vi "FPGA_frame.vi"(8 "error in":errorcluster) -> (0 "error out":errorcluster)   [LabVIEW 2010]
uses:
  fpgaVIsAndControls/DDS_board_init_cluster.ctl
  fpgaVIsAndControls/FPGA_parameters_cluster.ctl
  common_typedefs/channels_cluster.ctl
  fpgaVIsAndControls/scan_point_cluster.ctl
  common_typedefs/gate_parameters_cluster.ctl
  fpgaVIsAndControls/DDS_board_values_cluster.ctl
  fpgaVIsAndControls/synthesizer_point_cluster.ctl
  fpgaVIsAndControls/derived_values.ctl
  fpgaVIsAndControls/frame_scan_settings.ctl
  <vilib>/Platform/TimedLoop/XDataNode/XDataNode.xnode
  <vilib>/Platform/TimedLoop/XDataNode/timing_clust.ctl
  <vilib>/Platform/TimedLoop/XDataNode/nitl_modes.ctl
  <vilib>/Platform/TimedLoop/XDataNode/wakeup.ctl
  <vilib>/eio/EIONode/EIONode.xnode
  <vilib>/rvi/eio/nirviEIOImplementation/nirviEIOImplementation.xnode
  <vilib>/rvi/eio/common/nirviEmuClasses.ctl
  <vilib>/rvi/eio/nirviErrorMerge/nirviErrorMerge.xnode
  <vilib>/rvi/DataTransferAndStorage/Container/XNode/niFpgaContainer.xnode
  <vilib>/rvi/eio/common/nirviEmuTemplateMethod_noerrors.vi
  <vilib>/rvi/eio/common/nirviEmuTemplateMethod_errors.vi
  <vilib>/rvi/FIFO/Fifo_Resource/nirvififoEmulationSetSize.vi
  <vilib>/rvi/DataTransferAndStorage/Container/Common/niFpgaContainerGetUniqueNameForEmu.vi
  <vilib>/Platform/TimedLoop/XDataNode/XDNodeRunTimeDep.lvlib
panel:
  in  "shall acquisition start clocks?":bool
  in  "run clock 3":bool
  in  "run clock 2":bool
  in  "run clock 1":bool
  in  "scan settings":T1={"x-resolution"=10, "y-resolution"=10}
  out "derived values":T2={"AOD half bandwidth_x"=17500000.0, "AOD half bandwidth_y"=17500000.0, "x-point bandwidth"=10.0, "y-point bandwidth"=10.0} {"y-point bandwidth" format="%.28g"; "x-point bandwidth" format="%.28g"; "AOD half bandwidth_y" format="%.14g"; "AOD half bandwidth_x" format="%.14g"}
  in  "stop VI":bool
  out "synthesizer point out":T3
  out "frequency point":T4
  in  "clamp first pixel?":bool
  in  "gate 1":T5
  in  "gate 2":T5
  in  "gate 3":T5
  out "clock 2 state":bool
  out "clock 1 state":bool
  out "clock 3 state":bool
  out "acquiring?":bool
  in  "in triggered mode?":bool
  in  "stop at FIFO overflow?":bool
  in  "converter box version":i16=1 min=1 max=2
  out "current scan point":T6
  in  "amplitude":u16=3400
  in  "amp comp":bool
  out "reset out":bool
  in  "inverse?":T7(ring)
  in  "OSK select":bool=TRUE
  in  "FPGA parameters":T8={"AOD Bandwidth_x (Hz)"=34000000.0, "AOD Bandwidth_y (Hz)"=34000000.0, "sin Phi"=0.0, "cos Phi"=1.0, "Bandwidth for LUTs (256pts)"=0.9999999999854481, "AOD_Amplitude in"=3400, "AOD center frequ. (Hz)_x"=94000000.0, "AOD center frequ. (Hz)_y"=94000000.0, "x offset (Hz)"=0.0, "y offset (Hz)"=0.0} {"AOD center frequ. (Hz)_y" format="%.14g"; "AOD center frequ. (Hz)_x" format="%.14g"; "cos Phi" format="%.35g"; "sin Phi" format="%.35g"}
  out "integrated pixel values":T9
  in  "maximum bit depth":i8=16
  in  "intergration iterations per pixel":u32=40
  in  "waiting iterations  per pixel":u32=200
  out "data read":T9
  in  "channel offsets":T9
  in  "number of pixels":i64=-1
  out "FIFO_DMA full?":bool
  out "current pixel no.":i64
  out "current FPGA parameters":T8 {"AOD center frequ. (Hz)_y" format="%.14g"; "AOD center frequ. (Hz)_x" format="%.14g"; "cos Phi" format="%.35g"; "sin Phi" format="%.35g"}
  out "data sending counter (#bytes)":u32 caption="data sending counter"
  out "reset counter in":u8
  in  "acquire?":bool caption="Acquire?"
  in  "reset in":bool caption="Reset"
  in  "DDS board initialization parameters":T10={"Bypass PLL"=FALSE, "PLL Range"=TRUE, "Update Clock"=FALSE, "Triangle "=FALSE, "SDO Active"=FALSE, "LSB First"=FALSE, "OSK Int"=FALSE, "Output Shaped Keying Enable"=TRUE, "Bypass Sinc"=FALSE, "Digital Part"=TRUE, "OutPut DAC"=TRUE, "Control DAC"=FALSE, "Comparator"=FALSE, "Modus"=0, "Multiplier Value"=15} {"Modus" scale=0.0..4.0}
  # "FPGA integrator"
  # "Scan parameters"
  # "Clock parameters"
  # "DIO 1/32"
  # "CONFIG"
  # "PXI/RTSI 1"
  # "PXI/RTSI 2"
  # "Debug"
  # "FSK"
  # "Ramped"
  # "FSK"
  # "Chirp Modus"
  # "Unramped"
  # "BPSK"
  # "Single Tone"
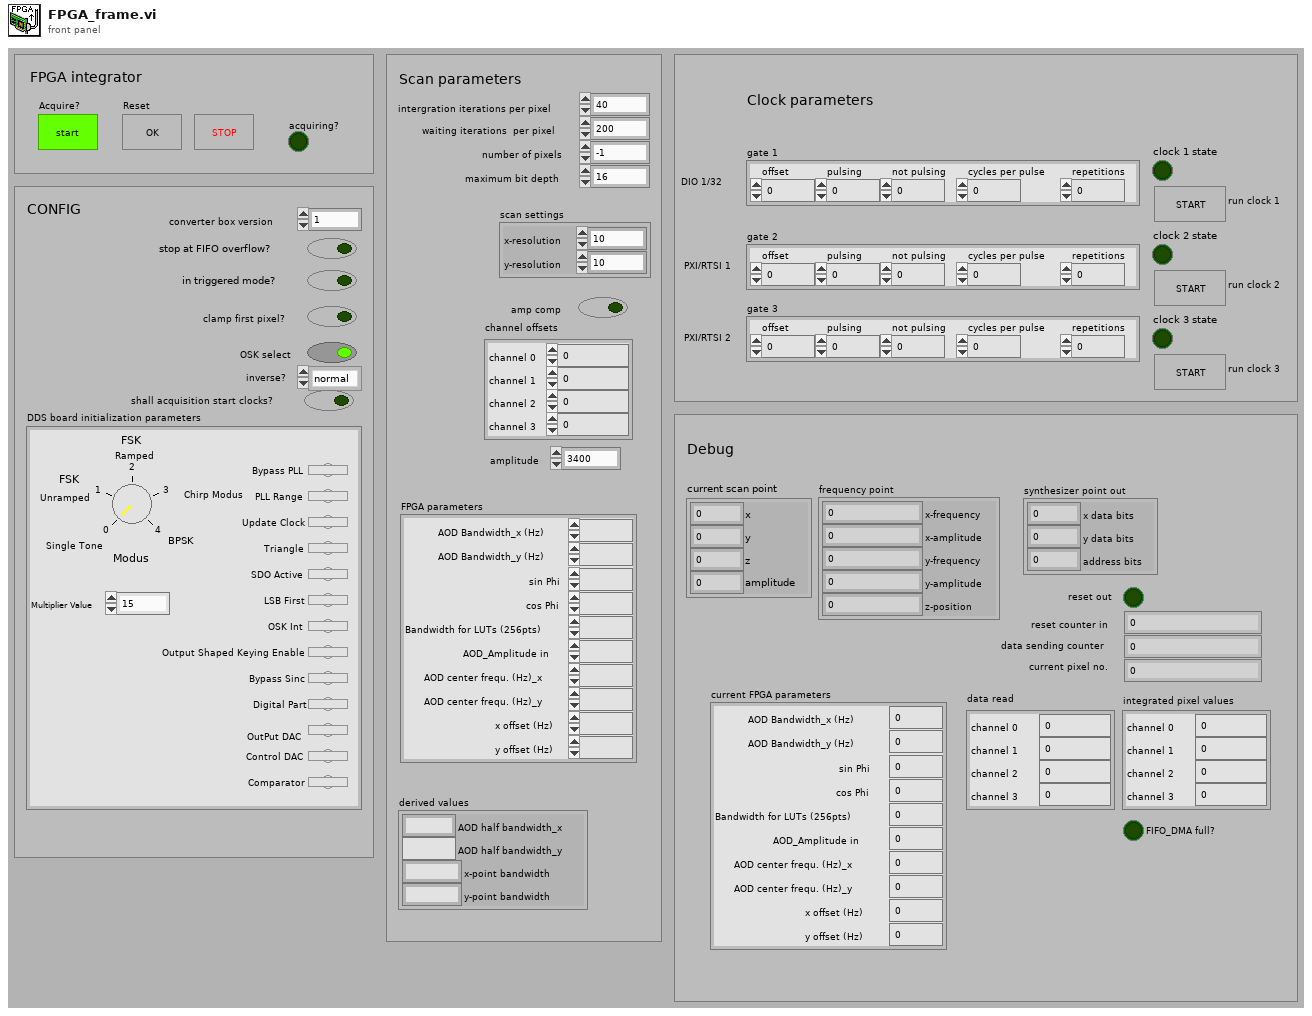
[diagram p1: front panel]
types:
  T1 = typedef "frame_scan_settings.ctl" = cluster{"x-resolution":u16, "y-resolution":u16}
  T2 = typedef "derived_values.ctl" = cluster{"AOD half bandwidth_x":fxp<+/-,36,32>, "AOD half bandwidth_y":fxp<+/-,36,32>, "x-point bandwidth":fxp<+/-,36,32>, "y-point bandwidth":fxp<+/-,36,32>}
  T3 = typedef "synthesizer_point_cluster.ctl" = cluster{"x data bits":u8, "y data bits":u8, "address bits":u8}
  T4 = typedef "DDS_board_values_cluster.ctl" = cluster{"x-frequency":fxp<+/-,36,32>, "x-amplitude":u16, "y-frequency":fxp<+/-,36,32>, "y-amplitude":u16, "z-position":i16}
  T5 = typedef "gate_parameters_cluster.ctl" = cluster{"offset":i64, "pulsing":i64, "not pulsing":i64, "cycles per pulse":i64, "repetitions":i64}
  T6 = typedef "scan_point_cluster.ctl" = cluster{"x":u16, "y":u16, "z":u16, "amplitude":u16}
  T7 = enum16{"normal", "x inversed", "y inversed", "x & y inversed"}
  T8 = typedef "FPGA_parameters_cluster.ctl" = cluster{"AOD Bandwidth_x (Hz)":fxp<+/-,36,32>, "AOD Bandwidth_y (Hz)":fxp<+/-,36,32>, "sin Phi":fxp<+/-,36,2>, "cos Phi":fxp<+/-,36,2>, "Bandwidth for LUTs (256pts)":fxp<+,36,0>, "AOD_Amplitude in":u16, "AOD center frequ. (Hz)_x":fxp<+/-,36,32>, "AOD center frequ. (Hz)_y":fxp<+/-,36,32>, "x offset (Hz)":fxp<+/-,36,32>, "y offset (Hz)":fxp<+/-,36,32>}
  T9 = typedef "channels_cluster.ctl" = cluster{"channel 0":u32, "channel 1":u32, "channel 2":u32, "channel 3":u32}
  T10 = typedef "DDS_board_init_cluster.ctl" = cluster{"Bypass PLL":bool, "PLL Range":bool, "Update Clock":bool, "Triangle ":bool, "SDO Active":bool, "LSB First":bool, "OSK Int":bool, "Output Shaped Keying Enable":bool, "Bypass Sinc":bool, "Digital Part":bool, "OutPut DAC":bool, "Control DAC":bool, "Comparator":bool, "Modus":u8, "Multiplier Value":u8}
  T11 = typedef "FPGA_constants_cluster.ctl" = cluster{"register":cluster{"Reg. 1D":u8, "Reg. 1E":u8, "Reg. 1F":u8, "Reg. 20":u8}}
  T12 = typedef "XDNodeRunTimeDep.lvlib/timing_clust.ctl" = cluster{"Expected End [f-1]":u64, "Actual End [f-1]":u64, "Finished Late? [f-1]":bool, "Expected End [i-1]":u64, "Actual End [i-1]":u64, "Finished Late? [i-1]":bool, "Expected Start [i]":u64, "Actual Start [i]":u64, "Expected Start [f]":u64, "Actual Start [f]":u64, "Source Name":string, "Structure Name":string, "Period":i64, "Deadline":i64, "Offset":i64, "Start":i64, "Priority":i32, "Timeout":i32, "Mode":T13, "Wakeup Reason":T14, "Error":errorcluster, "Source Type":string, "Secondary Source Type":string, "Global End Time":u64, "Global Start Time":u64, "Frame Duration":u64, "Iteration Duration":u64, "Assigned CPU":i32, "I/O Scan Engine Mode":u32}
  T13 = typedef "XDNodeRunTimeDep.lvlib/nitl_modes.ctl" = enum32{"No Change", "Process missed periods, maintain original phase", "Discard missed periods, maintain original phase", "Process missed periods, ignore original phase", "Discard missed periods, ignore original phase"}
  T14 = typedef "XDNodeRunTimeDep.lvlib/wakeup.ctl" = enum32{"Normal", "Aborted", "Asynchronous wakeup", "Timing source error", "Timed loop error", "Timeout"}
  T15 = typedef "nirviEmuClasses.ctl" = enum16{"IO Read", "IO Write", "Method", "Property Read", "Property Write"}
  T16 = typedef "gate_counters_cluster.ctl" = cluster{"phase iteration counter":i64, "phase repetition counter":i64, "pulse iteration counter":i64, "phase state":bool}
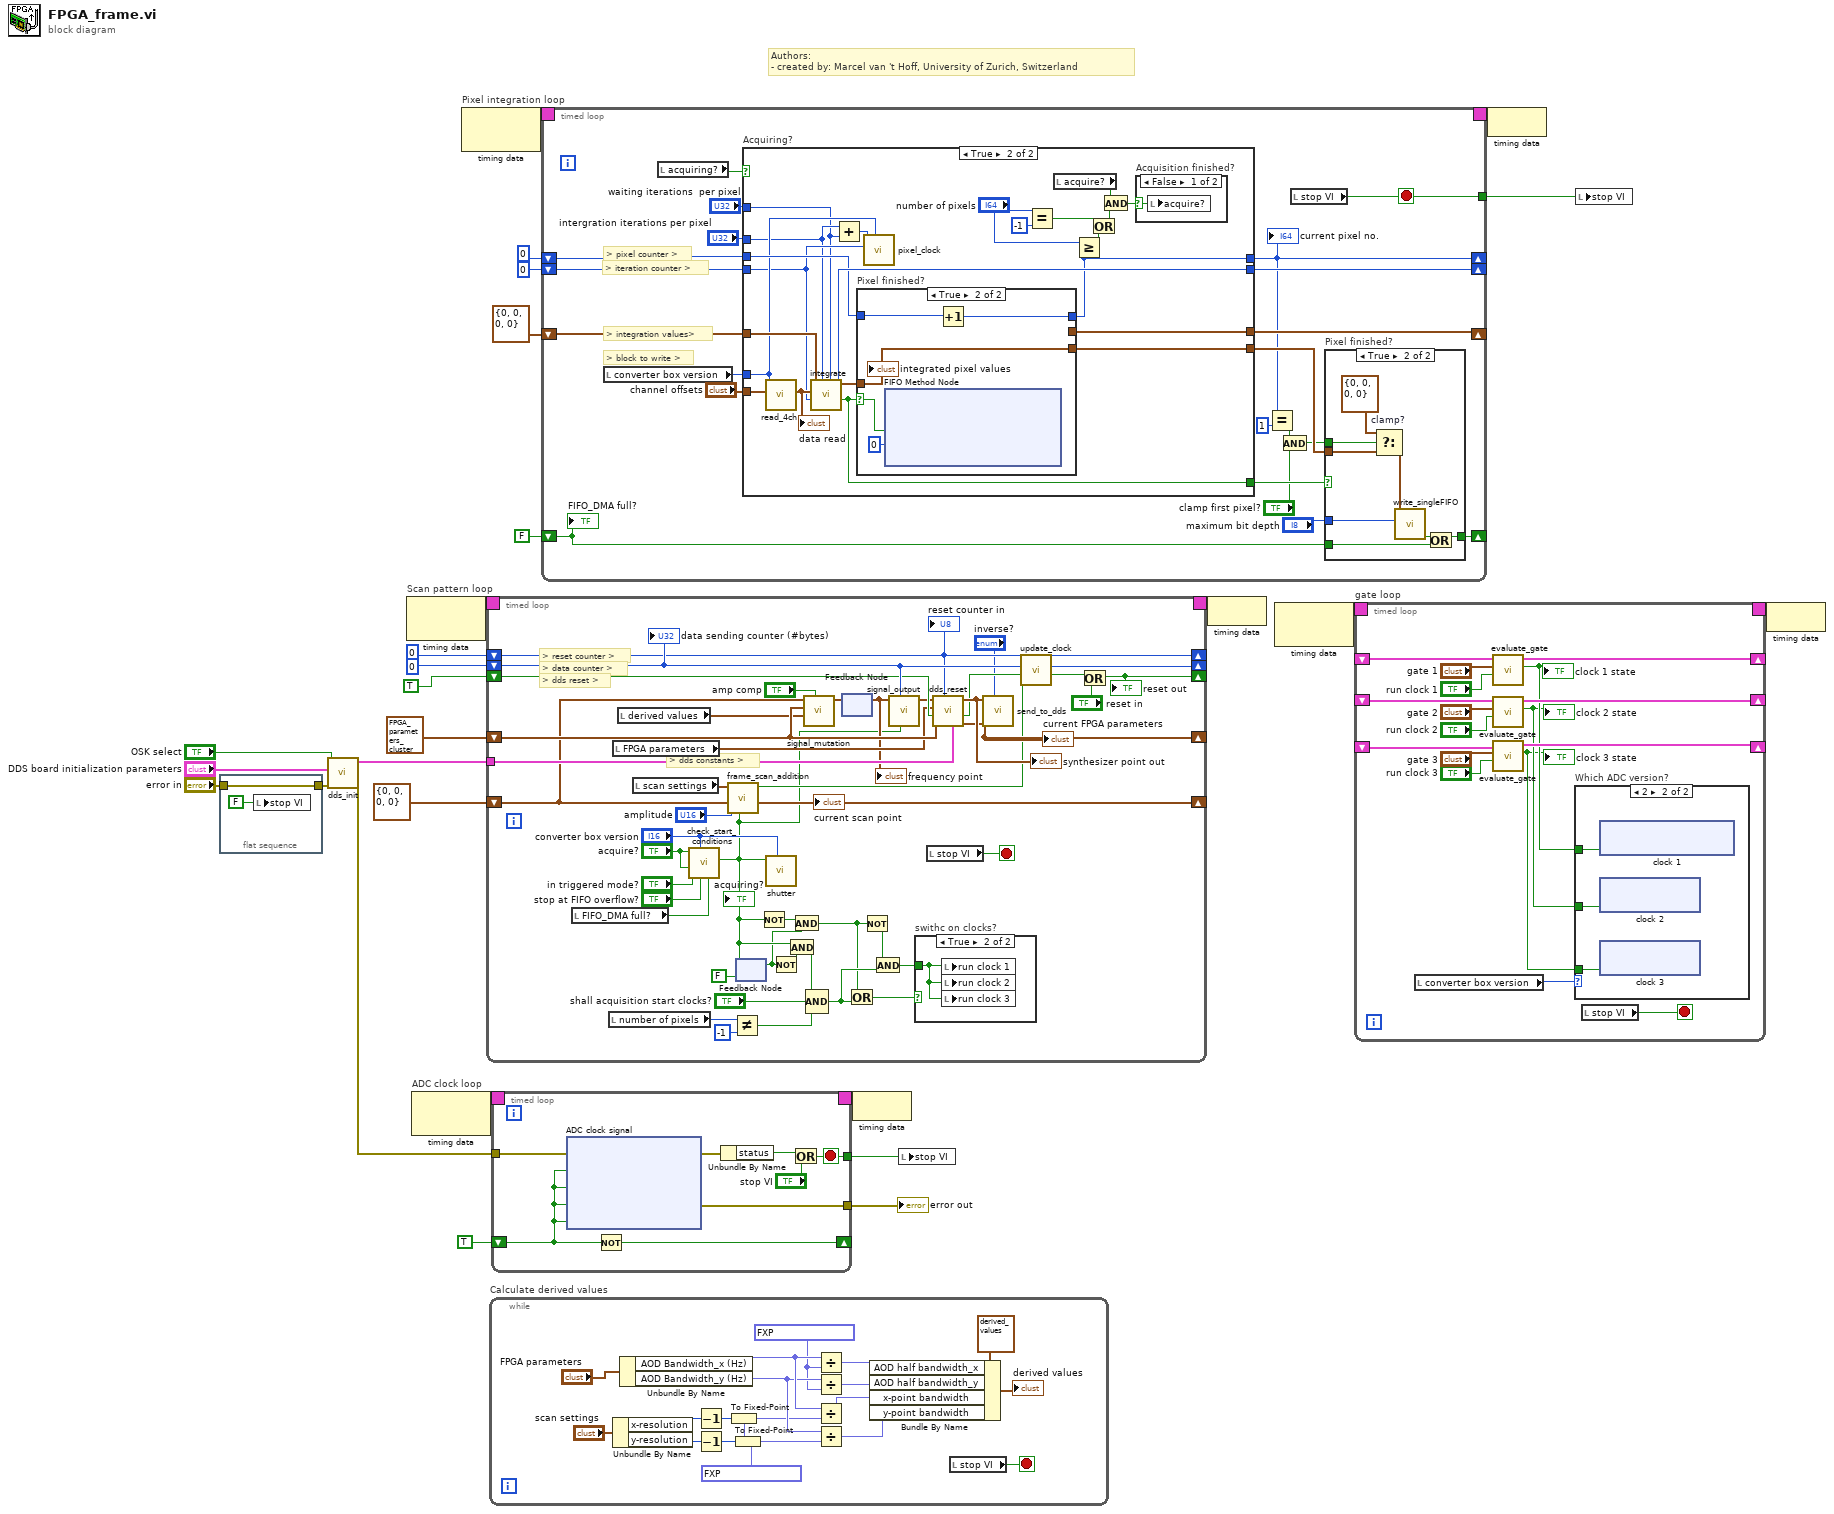
[diagram p0: block diagram]
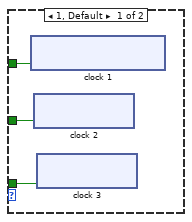
[diagram p2: hidden frame]
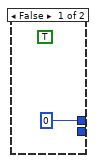
[diagram p5: hidden frame]
diagram:
  # "Authors: \n- created by: Marcel van 't Hoff, University of Zurich, Switzerland"
  n1 = flat-sequence {
    tunnel: "error in" -> [w28]
    tunnel: [w28] -> w1
    frame #0 {
      n2 = local write "stop VI"(FALSE ("stop VI")) -> ()
    }
  }
  n3 = call "dds_init.vi"("error in"=w1, "DDS board initialization parameters"="DDS board initialization parameters", "OSK select"="OSK select") -> ("error out"=w22:errorcluster, "constants out"=w23:T11)  [unwired: 7 in]
  n4 = node-c288() -> (w12:T12)  [unwired: 1 in]
  n5 = node-c288() -> (w27:T12)  [unwired: 1 out]
  n6 = node-c288() -> (w17:T12)  [unwired: 1 out]
  n7 = timed-loop "Scan pattern loop" {
    tunnel: w23 -> [w67]
    shift-right: [w64] -> _
    shift-left: T8 {"AOD Bandwidth_x (Hz)"=35000000.0, "AOD Bandwidth_y (Hz)"=35000000.0, "sin Phi"=1.9999999999417923, "cos Phi"=1.9999999999417923, "Bandwidth for LUTs (256pts)"=0.0, "AOD_Amplitude in"=0, "AOD center frequ. (Hz)_x"=1.0, "AOD center frequ. (Hz)_y"=0.0, "x offset (Hz)"=1.0, "y offset (Hz)"=0.0} ("FPGA parameters out 2") -> [w51]
    shift-right: [w73] -> _
    shift-left: TRUE ("reset dds out") -> [w62]
    shift-right: [w72] -> _
    shift-left: u32 0 ("data sending counter (#bytes)") -> [w71]
    shift-right: [w70] -> _
    shift-left: u8 0 ("reset counter in") -> [w66]
    timing: w12 -> [_]
    timing-out: [_] -> w11
    shift-right: [w50] -> _
    shift-left: T6 {"x"=0, "y"=0, "z"=0, "amplitude"=0} ("scan points cluster out") -> [w45]
    stop <- w74 stop-if-true
    # "> dds constants >"
    # "> data counter >"
    # "> reset counter >"
    # "> dds reset >"
    n8 = local read "FIFO_DMA full?"() -> (w58:bool)
    n9 = local read "number of pixels"() -> (w42:i64)
    n10 = local read "FPGA parameters"() -> (w49:T8)
    n11 = local read "derived values"() -> (w48:T2)
    n12 = local read "scan settings"() -> (w47:T1)
    n13 = call "check_start_conditions.vi"("FIFO overflow?"=w58, "stop at FIFO overflow?"="stop at FIFO overflow?", "converter box version"="converter box version", "already acquiring?"="acquire?", "in triggered mode?"="in triggered mode?", "acquire"="acquire?") -> ("acquire?"=w37:bool)  [unwired: 5 in]
    "acquiring?" <- w37
    n14 = call "frame_scan_addition.vi"("frame scanning?"=w37, "amplitude"="amplitude", "scan point"=w45, "scan settings"=w47) -> ("scan points cluster out"=w50:T6, "new pixel update?"=w63:bool)  [unwired: 6 in]
    "current scan point" <- w50
    n15 = Not Equal?(x=w42, y=i64 -1 ("x")) -> (x != y?=w41:bool)
    n16 = feedback-in #1(w37) -> ()
    n17 = feedback #1(FALSE ("acquire?")) -> (w35:bool)
    n18 = Not(x=w37) -> (.not. x?=w40:bool)
    n19 = call "shutter.vi"("converter box version"="converter box version", "open?"=w37) -> ()  [unwired: 10 in]
    n20 = Not(x=w35) -> (.not. x?=w38:bool)
    n21 = And(x=w37, y=w38) -> (x .and. y?=w36:bool)
    n22 = And(x=w40, y=w35) -> (x .and. y?=w30:bool)
    n23 = call "signal_mutation.vi"("amplitude compensation?"="amp comp", "derived values"=w48, "FPGA parameters"=w51, "point"=w45) -> ("frequency point"=w54:T4)  [unwired: 7 in]
    n24 = Compound Arithmetic op=AND(w36, "shall acquisition start clocks?", w41) -> (w32:bool)
    n25 = feedback-in #2(w54) -> ()
    n26 = feedback #2() -> (w46:T4)  [unwired: 1 in]
    "frequency point" <- w46
    n27 = Or(x=w30, y=w32) -> (x .or. y?=w33:bool)
    n28 = Not(x=w30) -> (.not. x?=w31:bool)
    n29 = And(x=w31, y=w32) -> (x .and. y?=w34:bool)
    n30 = call "signal_output.vi"("acquire?"=w37, "pipeline counter in"=w71, "frequency point"=w46) -> ("synthesizer point"=w52:T3)  [unwired: 8 in]
    n31 = case "swithc on clocks?" shown="True" w33 {
      tunnel: w34 -> [_ w76]
      frame False {
      }
      frame True {
        n32 = local write "run clock 1"(w76) -> ()
        n33 = local write "run clock 2"(w76) -> ()
        n34 = local write "run clock 3"(w76) -> ()
      }
    }
    n35 = local read "stop VI"() -> (w74:bool)
    n36 = call "dds_reset.vi"("constants in"=w67, "counter in"=w66, "FPGA parameters in"=w51, "reset dds in"=w62, "FPGA parameters after reset"=w49, "synthesizer point in"=w52) -> ("FPGA parameters out"=w64:T8, "reset dds out"=w69:bool, "synthesizer point out"=w75:T3)  [unwired: 3 in]
    "current FPGA parameters" <- w64
    "synthesizer point out" <- w75
    n37 = call "send_to_dds.vi"("inversion selector"="inverse?", "synthesizer point"=w75) -> ()  [unwired: 10 in]
    n38 = call "update_clock.vi"("update command in"=w63, "update reset counter in"=w69, "data sending counter (#bytes) in"=w71, "reset counter in"=w66) -> ("update reset counter out"=w65:bool, "data sending counter (#bytes) out"=w72:u32, "reset counter out"=w70:u8)  [unwired: 5 in]
    n39 = Or(x=w65, y="reset in") -> (x .or. y?=w73:bool)
    "reset out" <- w73
    "reset counter in" <- w66
    "data sending counter (#bytes)" <- w71
  }
  n40 = while "Calculate derived values" {
    stop <- w95 stop-if-true
    w79 = fxp<+/-,36,32> 2.0 ("y")
    w86 = fxp<+,36,32> 0.0 ("y")
    n41 = Unbundle By Name("scan settings") -> ("x-resolution"=w87:u16, "y-resolution"=w88:u16)
    n42 = Unbundle By Name("FPGA parameters") -> ("AOD Bandwidth_x (Hz)"=w92:fxp<+/-,36,32>, "AOD Bandwidth_y (Hz)"=w91:fxp<+/-,36,32>)
    n43 = Decrement(x=w87) -> (x-1=w85:u16)
    n44 = Decrement(x=w88) -> (x-1=w84:u16)
    n45 = To Fixed-Point(fixed-point type=w86, number=w85) -> (fixed-point=w90:fxp<+,36,32>)
    n46 = To Fixed-Point(fixed-point type=w86, number=w84) -> (fixed-point=w89:fxp<+,36,32>)
    n47 = Divide(x=w92, y=w79) -> (x/y=w94:fxp<+/-,36,32>)
    n48 = Divide(x=w91, y=w79) -> (x/y=w93:fxp<+/-,36,32>)
    n49 = Divide(x=w92, y=w90) -> (x/y=w81:fxp<+/-,36,32>)
    n50 = Divide(x=w91, y=w89) -> (x/y=w80:fxp<+/-,36,32>)
    n51 = Bundle By Name(cluster=T2 {"AOD half bandwidth_x"=17500000.0, "AOD half bandwidth_y"=17500000.0, "x-point bandwidth"=10.0, "y-point bandwidth"=10.0} ("derived values"), "AOD half bandwidth_x"=w94, "AOD half bandwidth_y"=w93, "x-point bandwidth"=w81, "y-point bandwidth"=w80) -> (→"derived values":T2)
    n52 = local read "stop VI"() -> (w95:bool)
  }
  n53 = timed-loop "ADC clock loop" {
    timing: w27 -> [_]
    timing-out: [_] -> w26
    shift-right: [w100] -> _
    shift-left: TRUE -> [w104]
    tunnel: [w102] -> w24
    tunnel: w22 -> [w101]
    tunnel: [w99] -> w9
    stop <- w102 stop-if-true
    n54 = xnode "ADC clock signal"("error in"=w101, "Connector0/DIO14"=w104, "Connector0/DIO15"=w104, "Connector1/DIO14"=w104, "Connector1/DIO15"=w104) -> ("error out"=w99:errorcluster)  [unwired: 4 in, 4 out]
    n55 = Not(x=w104) -> (.not. x?=w100:bool)
    n56 = Unbundle By Name(w99) -> ("status"=w103:bool)
    n57 = Or(x=w103, y="stop VI") -> (x .or. y?=w102:bool)
  }
  "error out" <- w9
  n58 = timed-loop "Pixel integration loop" {
    timing: w17 -> [_]
    timing-out: [_] -> w16
    shift-right: [w222] -> _
    shift-left: T9 {"channel 0"=0, "channel 1"=0, "channel 2"=0, "channel 3"=0} ("channel offsets 2") -> [w221]
    shift-right: [w219] -> _
    shift-left: u32 0 ("iteration counter out") -> [w220]
    shift-right: [w206] -> _
    shift-left: i64 0 -> [w218]
    tunnel: [w217] -> w13
    shift-right: [w202] -> _
    shift-left: FALSE -> [w203]
    stop <- w217 stop-if-true
    # "> pixel counter >"
    # "> block to write >"
    # "> integration values>"
    # "> iteration counter >"
    n59 = local read "converter box version"() -> (w213:i16)
    n60 = local read "acquiring?"() -> (w212:bool)
    n61 = case "Acquiring?" shown="True" w212 {
      tunnel: [_ w234] -> w222
      tunnel: w221 -> [_ w254]
      tunnel: [_ w241] -> w208
      tunnel: w220 -> [_ w239]
      tunnel: [_ w251] -> w219
      tunnel: w218 -> [_ w244]
      tunnel: [i64 0 w243] -> w206
      tunnel: "channel offsets" -> [_ w242]
      tunnel: "intergration iterations per pixel" -> [_ w237]
      tunnel: "waiting iterations  per pixel" -> [_ w236]
      tunnel: w213 -> [_ w240]
      tunnel: [_ w235] -> w211
      frame False {
        (unwired) TRUE
      }
      frame True {
        n62 = call "read_4ch.vi"("channel offsets"=w242, "converter box version"=w240) -> ("read output"=w252:T9)  [unwired: 9 in]
        "data read" <- w252
        n63 = call "integrate.vi"("waiting iterations per pixel"=w236, "integration iterations per pixel"=w237, "iteration counter in"=w239, "sampling values in"=w252, "previous pixel values in"=w254) -> ("finished?"=w235:bool, "iteration counter out"=w251:u32, "new pixel values out"=w253:T9)  [unwired: 4 in]
        n64 = Add(x=w237, y=w236) -> (x+y=w238:u32)
        n65 = case "Pixel finished?" shown="True" w235 {
          selector: w235 -> [_ w261]
          tunnel: w253 -> [w256 w262]
          tunnel: [_ w262] -> w241
          tunnel: w244 -> [w257 w259]
          tunnel: [w257 w258] -> w243
          tunnel: [w256 _] -> w234
          frame False {
          }
          frame True {
            n66 = xnode ("FIFO Method Node")("Element"=w261, "Timeout"=0) -> ()  [unwired: 1 in, 2 out]
            n67 = Increment(x=w259) -> (x+1=w258:i64)
            "integrated pixel values" <- w262
          }
        }
        n68 = call "pixel_clock.vi"("converter box version"=w240, "current iteration"=w239, "iterations per pixel"=w238) -> ()  [unwired: 9 in]
        n69 = Equal?(x="number of pixels", y=i64 -1 ("x")) -> (x = y?=w248:bool)
        n70 = local read "acquire?"() -> (w233:bool)
        n71 = Greater Or Equal?(x="number of pixels", y=w243) -> (x >= y?=w247:bool)
        n72 = Or(x=w248, y=w247) -> (x .or. y?=w249:bool)
        n73 = And(x=w233, y=w249) -> (x .and. y?=w250:bool)
        n74 = case "Acquisition finished?" shown="False" w250 {
          selector: w250 -> [w255 _]
          frame False {
            n75 = local write "acquire?"(w255) -> ()
          }
          frame True {
          }
        }
      }
    }
    "current pixel no." <- w206
    n76 = Equal?(x=w206, y=i64 1) -> (x = y?=w209:bool)
    n77 = And(x=w209, y="clamp first pixel?") -> (x .and. y?=w204:bool)
    n78 = local read "stop VI"() -> (w217:bool)
    n79 = case "Pixel finished?" shown="True" w211 {
      tunnel: w208 -> [_ w230]
      tunnel: "maximum bit depth" -> [_ w228]
      tunnel: w204 -> [_ w227]
      tunnel: w203 -> [w223 w225]
      tunnel: [w223 w224] -> w202
      frame False {
      }
      frame True {
        n80 = Select "clamp?"(t=T9 {"channel 0"=0, "channel 1"=0, "channel 2"=0, "channel 3"=0}, s=w227, f=w230) -> (s? t:f=w231:T9)
        n81 = call "write_singleFIFO.vi"("maximum bit depth"=w228, "values to be written"=w231) -> ("FIFO overflow"=w226:bool)  [unwired: 9 in]
        n82 = Or(x=w226, y=w225) -> (x .or. y?=w224:bool)
      }
    }
    "FIFO_DMA full?" <- w203
  }
  n83 = node-c288(w26) -> ()
  n84 = local write "stop VI"(w24) -> ()
  n85 = node-c288(w11) -> ()
  n86 = node-c288() -> (w4:T12)  [unwired: 1 in]
  n87 = timed-loop "gate loop" {
    timing: w4 -> [_]
    timing-out: [_] -> w3
    shift-right: [w331] -> _
    shift-left: _ -> [w332]
    shift-right: [w329] -> _
    shift-left: _ -> [w330]
    shift-right: [w328] -> _
    shift-left: _ -> [w327]
    stop <- w319 stop-if-true
    n88 = local read "converter box version"() -> (w320:i16)
    n89 = call "evaluate_gate.vi"("acquiring?"="run clock 1", "gate settings"="gate 1", "gate counters in"=w332) -> ("pulse state out"=w323:bool, "gate counters out"=w331:T16)  [unwired: 7 in]
    "clock 1 state" <- w323
    n90 = call "evaluate_gate.vi"("acquiring?"="run clock 2", "gate settings"="gate 2", "gate counters in"=w330) -> ("pulse state out"=w322:bool, "gate counters out"=w329:T16)  [unwired: 7 in]
    "clock 2 state" <- w322
    n91 = call "evaluate_gate.vi"("acquiring?"="run clock 3", "gate settings"="gate 3", "gate counters in"=w327) -> ("pulse state out"=w321:bool, "gate counters out"=w328:T16)  [unwired: 7 in]
    "clock 3 state" <- w321
    n92 = case "Which ADC version?" shown="2" w320 {
      tunnel: w323 -> [w333 w371]
      tunnel: w322 -> [w334 w370]
      tunnel: w321 -> [w335 w369]
      frame 1, Default {
        n93 = xnode "clock 1"("Connector1/DIO32"=w333) -> ()  [unwired: 1 in, 1 out]
        n94 = xnode "clock 2"("PXI_RTSI_1"=w334) -> ()  [unwired: 1 in, 1 out]
        n95 = xnode "clock 3"("PXI_RTSI_2"=w335) -> ()  [unwired: 1 in, 1 out]
      }
      frame 2 {
        n96 = xnode "clock 1"("Connector0/DIO38"=w371) -> ()  [unwired: 1 in, 1 out]
        n97 = xnode "clock 2"("PXI_RTSI_1"=w370) -> ()  [unwired: 1 in, 1 out]
        n98 = xnode "clock 3"("PXI_RTSI_2"=w369) -> ()  [unwired: 1 in, 1 out]
      }
    }
    n99 = local read "stop VI"() -> (w319:bool)
  }
  n100 = node-c288(w16) -> ()
  n101 = local write "stop VI"(w13) -> ()
  n102 = node-c288(w3) -> ()
